vi "Weather Parse Test.vi"() -> ()   [LabVIEW 2020, in "CDM-Config.lvlib"] (continued)
        \"properties\": {\n                \"@id\": \"https://api.weather.gov/alerts/urn:oid:2.49.0.1.840.0.3fac73b358a1e250101ceb2ba749b5bee3a29f80.005.1\",\n                \"@type\": \"wx:Alert\",\n                \"id\": \"urn:oid:2.49.0.1.840.0.3fac73b358a1e250101ceb2ba749b5bee3a29f80.005.1\",\n                \"areaDesc\": \"Cape Cleare to Gore Point out to 15 NM\",\n                \"geocode\": {\n                    \"SAME\": [\n                        \"058715\"\n                    ],\n                    \"UGC\": [\n                        \"PKZ715\"\n                    ]\n                },\n                \"affectedZones\": [\n                    \"https://api.weather.gov/zones/forecast/PKZ715\"\n                ],\n                \"references\": [],\n                \"sent\": \"2025-12-03T04:02:00-09:00\",\n                \"effective\": \"2025-12-03T04:02:00-09:00\",\n                \"onset\": \"2025-12-03T04:00:00-09:00\",\n                \"expires\": \"2025-12-03T16:30:00-09:00\",\n                \"ends\": \"2025-12-04T05:00:00-09:00\",\n                \"status\": \"Actual\",\n                \"messageType\": \"Alert\",\n                \"category\": \"Met\",\n                \"severity\": \"Minor\",\n                \"certainty\": \"Likely\",\n                \"urgency\": \"Expected\",\n                \"event\": \"Small Craft Advisory\",\n                \"sender\": \"w-nws.webmaster@noaa.gov\",\n                \"senderName\": \"NWS Anchorage AK\",\n                \"headline\": \"Small Craft Advisory issued December 3 at 4:02AM AKST until December 4 at 5:00AM AKST by NWS Anchorage AK\",\n                \"description\": \"Coastal Waters Forecast for the Northern Gulf of Alaska Coast\\nup to 100 nm out including Kodiak Island and Cook Inlet.\\n\\nWind forecasts reflect the predominant speed and direction\\nexpected. Sea forecasts represent an average of the highest\\none-third of the combined wind wave and swell height.\\n\\n.TODAY...Variable wind 10 kt. Seas 8 ft. Rain.\\n.TONIGHT...Variable wind 10 kt. Seas 8 ft.\\n.THU...Variable wind 10 kt. Seas 7 ft.\\n.THU NIGHT...Variable wind 10 kt. Seas 6 ft.\\n.FRI...N wind 20 kt. Seas 5 ft.\\n.SAT THROUGH SUN...NE wind 25 kt. Seas 9 ft.\",\n                \"instruction\": null,\n                \"response\": \"Avoid\",\n                \"parameters\": {\n                    \"AWIPSidentifier\": [\n                        \"CWFAER\"\n                    ],\n                    \"WMOidentifier\": [\n                        \"FZAK51 PAFC 031302\"\n                    ],\n                    \"NWSheadline\": [\n                        \"SMALL CRAFT ADVISORY THROUGH TONIGHT\"\n                    ],\n                    \"BLOCKCHANNEL\": [\n                        \"EAS\",\n                        \"NWEM\",\n                        \"CMAS\"\n                    ],\n                    \"VTEC\": [\n                        \"/O.NEW.PAFC.SC.Y.9733.251203T1300Z-251204T1400Z/\"\n                    ],\n                    \"eventEndingTime\": [\n                        \"2025-12-04T05:00:00-09:00\"\n                    ]\n                },\n                \"scope\": \"Public\",\n                \"code\": \"IPAWSv1.0\",\n                \"language\": \"en-US\",\n                \"web\": \"http://www.weather.gov\",\n                \"eventCode\": {\n                    \"SAME\": [\n                        \"NWS\"\n                    ],\n                    \"NationalWeatherService\": [\n                        \"SCY\"\n                    ]\n                }\n            }\n        },\n        {\n            \"id\": \"https://api.weather.gov/alerts/urn:oid:2.49.0.1.840.0.3fac73b358a1e250101ceb2ba749b5bee3a29f80.004.1\",\n            \"type\": \"Feature\",\n            \"geometry\": null,\n            \"properties\": {\n                \"@id\": \"https://api.weather.gov/alerts/urn:oid:2.49.0.1.840.0.3fac73b358a1e250101ceb2ba749b5bee3a29f80.004.1\",\n                \"@type\": \"wx:Alert\",\n                \"id\": \"urn:oid:2.49.0.1.840.0.3fac73b358a1e250101ceb2ba749b5bee3a29f80.004.1\",\n                \"areaDesc\": \"Cape Suckling to Cape Cleare from 15 to 75 NM\",\n                \"geocode\": {\n                    \"SAME\": [\n                        \"058712\"\n                    ],\n                    \"UGC\": [\n                        \"PKZ712\"\n                    ]\n                },\n                \"affectedZones\": [\n                    \"https://api.weather.gov/zones/forecast/PKZ712\"\n                ],\n                \"references\": [],\n                \"sent\": \"2025-12-03T04:02:00-09:00\",\n                \"effective\": \"2025-12-03T04:02:00-09:00\",\n                \"onset\": \"2025-12-03T04:00:00-09:00\",\n                \"expires\": \"2025-12-03T16:30:00-09:00\",\n                \"ends\": \"2025-12-04T17:00:00-09:00\",\n                \"status\": \"Actual\",\n                \"messageType\": \"Alert\",\n                \"category\": \"Met\",\n                \"severity\": \"Minor\",\n                \"certainty\": \"Likely\",\n                \"urgency\": \"Expected\",\n                \"event\": \"Small Craft Advisory\",\n                \"sender\": \"w-nws.webmaster@noaa.gov\",\n                \"senderName\": \"NWS Anchorage AK\",\n                \"headline\": \"Small Craft Advisory issued December 3 at 4:02AM AKST until December 4 at 5:00PM AKST by NWS Anchorage AK\",\n                \"description\": \"Coastal Waters Forecast for the Northern Gulf of Alaska Coast\\nup to 100 nm out including Kodiak Island and Cook Inlet.\\n\\nWind forecasts reflect the predominant speed and direction\\nexpected. Sea forecasts represent an average of the highest\\none-third of the combined wind wave and swell height.\\n\\n.TODAY...S wind 15 kt. Seas 11 ft.\\n.TONIGHT...SW wind 15 kt. Seas 10 ft.\\n.THU...SW wind 15 kt. Seas 9 ft.\\n.THU NIGHT...Variable wind 10 kt. Seas 8 ft.\\n.FRI...N wind 15 kt. Seas 7 ft.\\n.SAT...SE wind 25 kt. Seas 9 ft.\\n.SUN...E wind 25 kt. Seas 13 ft.\",\n                \"instruction\": null,\n                \"response\": \"Avoid\",\n                \"parameters\": {\n                    \"AWIPSidentifier\": [\n                        \"CWFAER\"\n                    ],\n                    \"WMOidentifier\": [\n                        \"FZAK51 PAFC 031302\"\n                    ],\n                    \"NWSheadline\": [\n                        \"SMALL CRAFT ADVISORY THROUGH THURSDAY\"\n                    ],\n                    \"BLOCKCHANNEL\": [\n                        \"EAS\",\n                        \"NWEM\",\n                        \"CMAS\"\n                    ],\n                    \"VTEC\": [\n                        \"/O.NEW.PAFC.SC.Y.9732.251203T1300Z-251205T0200Z/\"\n                    ],\n                    \"eventEndingTime\": [\n                        \"2025-12-04T17:00:00-09:00\"\n                    ]\n                },\n                \"scope\": \"Public\",\n                \"code\": \"IPAWSv1.0\",\n                \"language\": \"en-US\",\n                \"web\": \"http://www.weather.gov\",\n                \"eventCode\": {\n                    \"SAME\": [\n                        \"NWS\"\n                    ],\n                    \"NationalWeatherService\": [\n                        \"SCY\"\n                    ]\n                }\n            }\n        },\n        {\n            \"id\": \"https://api.weather.gov/alerts/urn:oid:2.49.0.1.840.0.3fac73b358a1e250101ceb2ba749b5bee3a29f80.017.1\",\n            \"type\": \"Feature\",\n            \"geometry\": null,\n            \"properties\": {\n                \"@id\": \"https://api.weather.gov/alerts/urn:oid:2.49.0.1.840.0.3fac73b358a1e250101ceb2ba749b5bee3a29f80.017.1\",\n                \"@type\": \"wx:Alert\",\n                \"id\": \"urn:oid:2.49.0.1.840.0.3fac73b358a1e250101ceb2ba749b5bee3a29f80.017.1\",\n                \"areaDesc\": \"Gore Point to Marmot Island from 15 to 80 NM\",\n                \"geocode\": {\n                    \"SAME\": [\n                        \"058733\"\n                    ],\n                    \"UGC\": [\n                        \"PKZ733\"\n                    ]\n                },\n                \"affectedZones\": [\n                    \"https://api.weather.gov/zones/forecast/PKZ733\"\n                ],\n                \"references\": [],\n                \"sent\": \"2025-12-03T04:02:00-09:00\",\n                \"effective\": \"2025-12-03T04:02:00-09:00\",\n                \"onset\": \"2025-12-03T04:00:00-09:00\",\n                \"expires\": \"2025-12-03T16:30:00-09:00\",\n                \"ends\": \"2025-12-04T17:00:00-09:00\",\n                \"status\": \"Actual\",\n                \"messageType\": \"Alert\",\n                \"category\": \"Met\",\n                \"severity\": \"Minor\",\n                \"certainty\": \"Likely\",\n                \"urgency\": \"Expected\",\n                \"event\": \"Small Craft Advisory\",\n                \"sender\": \"w-nws.webmaster@noaa.gov\",\n                \"senderName\": \"NWS Anchorage AK\",\n                \"headline\": \"Small Craft Advisory issued December 3 at 4:02AM AKST until December 4 at 5:00PM AKST by NWS Anchorage AK\",\n                \"description\": \"Coastal Waters Forecast for the Northern Gulf of Alaska Coast\\nup to 100 nm out including Kodiak Island and Cook Inlet.\\n\\nWind forecasts reflect the predominant speed and direction\\nexpected. Sea forecasts represent an average of the highest\\none-third of the combined wind wave and swell height.\\n\\n.TODAY...SW wind 20 kt. Seas 11 ft.\\n.TONIGHT...SW wind 15 kt. Seas 10 ft.\\n.THU...S wind 15 kt. Seas 8 ft.\\n.THU NIGHT...Variable wind 10 kt. Seas 7 ft.\\n.FRI...N wind 25 kt. Seas 7 ft.\\n.SAT...N wind 25 kt. Seas 11 ft.\\n.SUN...NE wind 25 kt. Seas 16 ft.\",\n                \"instruction\": null,\n                \"response\": \"Avoid\",\n                \"parameters\": {\n                    \"AWIPSidentifier\": [\n                        \"CWFAER\"\n                    ],\n                    \"WMOidentifier\": [\n                        \"FZAK51 PAFC 031302\"\n                    ],\n                    \"NWSheadline\": [\n                        \"SMALL CRAFT ADVISORY THROUGH THURSDAY\"\n                    ],\n                    \"BLOCKCHANNEL\": [\n                        \"EAS\",\n                        \"NWEM\",\n                        \"CMAS\"\n                    ],\n                    \"VTEC\": [\n                        \"/O.NEW.PAFC.SC.Y.9735.251203T1300Z-251205T0200Z/\"\n                    ],\n                    \"eventEndingTime\": [\n                        \"2025-12-04T17:00:00-09:00\"\n                    ]\n                },\n                \"scope\": \"Public\",\n                \"code\": \"IPAWSv1.0\",\n                \"language\": \"en-US\",\n                \"web\": \"http://www.weather.gov\",\n                \"eventCode\": {\n                    \"SAME\": [\n                        \"NWS\"\n                    ],\n                    \"NationalWeatherService\": [\n                        \"SCY\"\n                    ]\n                }\n            }\n        },\n        {\n            \"id\": \"https://api.weather.gov/alerts/urn:oid:2.49.0.1.840.0.3fac73b358a1e250101ceb2ba749b5bee3a29f80.006.1\",\n            \"type\": \"Feature\",\n            \"geometry\": null,\n            \"properties\": {\n                \"@id\": \"https://api.weather.gov/alerts/urn:oid:2.49.0.1.840.0.3fac73b358a1e250101ceb2ba749b5bee3a29f80.006.1\",\n                \"@type\": \"wx:Alert\",\n                \"id\": \"urn:oid:2.49.0.1.840.0.3fac73b358a1e250101ceb2ba749b5bee3a29f80.006.1\",\n                \"areaDesc\": \"Cape Cleare to Gore Point from 15 to 75 NM\",\n                \"geocode\": {\n                    \"SAME\": [\n                        \"058716\"\n                    ],\n                    \"UGC\": [\n                        \"PKZ716\"\n                    ]\n                },\n                \"affectedZones\": [\n                    \"https://api.weather.gov/zones/forecast/PKZ716\"\n                ],\n                \"references\": [],\n                \"sent\": \"2025-12-03T04:02:00-09:00\",\n                \"effective\": \"2025-12-03T04:02:00-09:00\",\n                \"onset\": \"2025-12-03T04:00:00-09:00\",\n                \"expires\": \"2025-12-03T16:30:00-09:00\",\n                \"ends\": \"2025-12-04T17:00:00-09:00\",\n                \"status\": \"Actual\",\n                \"messageType\": \"Alert\",\n                \"category\": \"Met\",\n                \"severity\": \"Minor\",\n                \"certainty\": \"Likely\",\n                \"urgency\": \"Expected\",\n                \"event\": \"Small Craft Advisory\",\n                \"sender\": \"w-nws.webmaster@noaa.gov\",\n                \"senderName\": \"NWS Anchorage AK\",\n                \"headline\": \"Small Craft Advisory issued December 3 at 4:02AM AKST until December 4 at 5:00PM AKST by NWS Anchorage AK\",\n                \"description\": \"Coastal Waters Forecast for the Northern Gulf of Alaska Coast\\nup to 100 nm out including Kodiak Island and Cook Inlet.\\n\\nWind forecasts reflect the predominant speed and direction\\nexpected. Sea forecasts represent an average of the highest\\none-third of the combined wind wave and swell height.\\n\\n.TODAY...SW wind 15 kt. Seas 10 ft.\\n.TONIGHT...SW wind 15 kt. Seas 10 ft.\\n.THU...SW wind 15 kt. Seas 8 ft.\\n.THU NIGHT...Variable wind 10 kt. Seas 7 ft.\\n.FRI...N wind 15 kt. Seas 7 ft.\\n.SAT...NE wind 25 kt. Seas 11 ft.\\n.SUN...NE wind 25 kt. Seas 15 ft.\",\n                \"instruction\": null,\n                \"response\": \"Avoid\",\n                \"parameters\": {\n                    \"AWIPSidentifier\": [\n                        \"CWFAER\"\n                    ],\n                    \"WMOidentifier\": [\n                        \"FZAK51 PAFC 031302\"\n                    ],\n                    \"NWSheadline\": [\n                        \"SMALL CRAFT ADVISORY THROUGH THURSDAY\"\n                    ],\n                    \"BLOCKCHANNEL\": [\n                        \"EAS\",\n                        \"NWEM\",\n                        \"CMAS\"\n                    ],\n                    \"VTEC\": [\n                        \"/O.NEW.PAFC.SC.Y.9734.251203T1300Z-251205T0200Z/\"\n                    ],\n                    \"eventEndingTime\": [\n                        \"2025-12-04T17:00:00-09:00\"\n                    ]\n                },\n                \"scope\": \"Public\",\n                \"code\": \"IPAWSv1.0\",\n                \"language\": \"en-US\",\n                \"web\": \"http://www.weather.gov\",\n                \"eventCode\": {\n                    \"SAME\": [\n                        \"NWS\"\n                    ],\n                    \"NationalWeatherService\": [\n                        \"SCY\"\n                    ]\n                }\n            }\n        },\n        {\n            \"id\": \"https://api.weather.gov/alerts/urn:oid:2.49.0.1.840.0.3fac73b358a1e250101ceb2ba749b5bee3a29f80.002.1\",\n            \"type\": \"Feature\",\n            \"geometry\": null,\n            \"properties\": {\n                \"@id\": \"https://api.weather.gov/alerts/urn:oid:2.49.0.1.840.0.3fac73b358a1e250101ceb2ba749b5bee3a29f80.002.1\",\n                \"@type\": \"wx:Alert\",\n                \"id\": \"urn:oid:2.49.0.1.840.0.3fac73b358a1e250101ceb2ba749b5bee3a29f80.002.1\",\n                \"areaDesc\": \"Cape Suckling to Gravel Point out to 15 NM\",\n                \"geocode\": {\n                    \"SAME\": [\n                        \"058710\"\n                    ],\n                    \"UGC\": [\n                        \"PKZ710\"\n                    ]\n                },\n                \"affectedZones\": [\n                    \"https://api.weather.gov/zones/forecast/PKZ710\"\n                ],\n                \"references\": [],\n                \"sent\": \"2025-12-03T04:02:00-09:00\",\n                \"effective\": \"2025-12-03T04:02:00-09:00\",\n                \"onset\": \"2025-12-03T04:00:00-09:00\",\n                \"expires\": \"2025-12-03T16:30:00-09:00\",\n                \"ends\": \"2025-12-04T17:00:00-09:00\",\n                \"status\": \"Actual\",\n                \"messageType\": \"Alert\",\n                \"category\": \"Met\",\n                \"severity\": \"Minor\",\n                \"certainty\": \"Likely\",\n                \"urgency\": \"Expected\",\n                \"event\": \"Small Craft Advisory\",\n                \"sender\": \"w-nws.webmaster@noaa.gov\",\n                \"senderName\": \"NWS Anchorage AK\",\n                \"headline\": \"Small Craft Advisory issued December 3 at 4:02AM AKST until December 4 at 5:00PM AKST by NWS Anchorage AK\",\n                \"description\": \"Coastal Waters Forecast for the Northern Gulf of Alaska Coast\\nup to 100 nm out including Kodiak Island and Cook Inlet.\\n\\nWind forecasts reflect the predominant speed and direction\\nexpected. Sea forecasts represent an average of the highest\\none-third of the combined wind wave and swell height.\\n\\n.TODAY...SE wind 25 kt becoming S 15 kt in the afternoon.\\nSeas 10 ft. Rain.\\n.TONIGHT...SW wind 15 kt. Seas 9 ft.\\n.THU...Variable wind 10 kt. Seas 8 ft.\\n.THU NIGHT...Variable wind 10 kt. Seas 7 ft.\\n.FRI...NE wind 25 kt. Seas 6 ft.\\n.SAT THROUGH SUN...NE wind 30 kt. Seas 9 ft.\",\n                \"instruction\": null,\n                \"response\": \"Avoid\",\n                \"parameters\": {\n                    \"AWIPSidentifier\": [\n                        \"CWFAER\"\n                    ],\n                    \"WMOidentifier\": [\n                        \"FZAK51 PAFC 031302\"\n                    ],\n                    \"NWSheadline\": [\n                        \"SMALL CRAFT ADVISORY THROUGH THURSDAY\"\n                    ],\n                    \"BLOCKCHANNEL\": [\n                        \"EAS\",\n                        \"NWEM\",\n                        \"CMAS\"\n                    ],\n                    \"VTEC\": [\n                        \"/O.NEW.PAFC.SC.Y.9730.251203T1300Z-251205T0200Z/\"\n                    ],\n                    \"eventEndingTime\": [\n                        \"2025-12-04T17:00:00-09:00\"\n                    ]\n                },\n                \"scope\": \"Public\",\n                \"code\": \"IPAWSv1.0\",\n                \"language\": \"en-US\",\n                \"web\": \"http://www.weather.gov\",\n                \"eventCode\": {\n                    \"SAME\": [\n                        \"NWS\"\n                    ],\n                    \"NationalWeatherService\": [\n                        \"SCY\"\n                    ]\n                }\n            }\n        },\n        {\n            \"id\": \"https://api.weather.gov/alerts/urn:oid:2.49.0.1.840.0.16ee1729296b80b5948b72c512c8722f6075ae6c.004.1\",\n            \"type\": \"Feature\",\n            \"geometry\": null,\n            \"properties\": {\n                \"@id\": \"https://api.weather.gov/alerts/urn:oid:2.49.0.1.840.0.16ee1729296b80b5948b72c512c8722f6075ae6c.004.1\",\n                \"@type\": \"wx:Alert\",\n                \"id\": \"urn:oid:2.49.0.1.840.0.16ee1729296b80b5948b72c512c8722f6075ae6c.004.1\",\n                \"areaDesc\": \"Castle Cape to Cape Tolstoi out to 15 NM\",\n                \"geocode\": {\n                    \"SAME\": [\n                        \"058752\"\n                    ],\n                    \"UGC\": [\n                        \"PKZ752\"\n                    ]\n                },\n                \"affectedZones\": [\n                    \"https://api.weather.gov/zones/forecast/PKZ752\"\n                ],\n                \"references\": [],\n                \"sent\": \"2025-12-03T04:00:00-09:00\",\n                \"effective\": \"2025-12-03T04:00:00-09:00\",\n                \"onset\": \"2025-12-03T04:00:00-09:00\",\n                \"expires\": \"2025-12-03T17:00:00-09:00\",\n                \"ends\": \"2025-12-04T17:00:00-09:00\",\n                \"status\": \"Actual\",\n                \"messageType\": \"Alert\",\n                \"category\": \"Met\",\n                \"severity\": \"Minor\",\n                \"certainty\": \"Likely\",\n                \"urgency\": \"Expected\",\n                \"event\": \"Small Craft Advisory\",\n                \"sender\": \"w-nws.webmaster@noaa.gov\",\n                \"senderName\": \"NWS Anchorage AK\",\n                \"headline\": \"Small Craft Advisory issued December 3 at 4:00AM AKST until December 4 at 5:00PM AKST by NWS Anchorage AK\",\n                \"description\": \"Coastal Waters Forecast for Southwest Alaska+Bristol Bay+The\\nAlaska Peninsula Waters and the Aleutian Islands up to 100 nm out.\\n\\nWind forecasts reflect the predominant speed and direction\\nexpected. Sea forecasts represent an average of the highest\\none-third of the combined wind wave and swell height.\\n\\n.TODAY...SE wind 20 kt. Seas 9 ft. Rain showers.\\n.TONIGHT...SE wind 20 kt. Seas 9 ft. Rain showers.\\n.THU...SE wind 15 kt. Seas 8 ft. Rain showers.\\n.THU NIGHT...NE wind 20 kt. Seas 6 ft.\\n.FRI...N wind 20 kt. Seas 5 ft.\\n.SAT...NW wind 35 kt. Seas 5 ft.\\n.SUN...N wind 20 kt. Seas 2 ft.\",\n                \"instruction\": null,\n                \"response\": \"Avoid\",\n                \"parameters\": {\n                    \"AWIPSidentifier\": [\n                        \"CWFALU\"\n                    ],\n                    \"WMOidentifier\": [\n                        \"FZAK52 PAFC 031300\"\n                    ],\n                    \"NWSheadline\": [\n                        \"SMALL CRAFT ADVISORY THROUGH THURSDAY\"\n                    ],\n                    \"BLOCKCHANNEL\": [\n                        \"EAS\",\n                        \"NWEM\",\n                        \"CMAS\"\n                    ],\n                    \"VTEC\": [\n                        \"/O.NEW.PAFC.SC.Y.5640.251203T1300Z-251205T0200Z/\"\n                    ],\n                    \"eventEndingTime\": [\n                        \"2025-12-04T17:00:00-09:00\"\n                    ]\n                },\n                \"scope\": \"Public\",\n                \"code\": \"IPAWSv1.0\",\n                \"language\": \"en-US\",\n                \"web\": \"http://www.weather.gov\",\n                \"eventCode\": {\n                    \"SAME\": [\n                        \"NWS\"\n                    ],\n                    \"NationalWeatherService\": [\n                        \"SCY\"\n                    ]\n                }\n            }\n        },\n        {\n            \"id\": \"https://api.weather.gov/alerts/urn:oid:2.49.0.1.840.0.16ee1729296b80b5948b72c512c8722f6075ae6c.003.1\",\n            \"type\": \"Feature\",\n            \"geometry\": null,\n            \"properties\": {\n                \"@id\": \"https://api.weather.gov/alerts/urn:oid:2.49.0.1.840.0.16ee1729296b80b5948b72c512c8722f6075ae6c.003.1\",\n                \"@type\": \"wx:Alert\",\n                \"id\": \"urn:oid:2.49.0.1.840.0.16ee1729296b80b5948b72c512c8722f6075ae6c.003.1\",\n                \"areaDesc\": \"Sitkinak to Castle Cape from 15 to 100 NM\",\n                \"geocode\": {\n                    \"SAME\": [\n                        \"058751\"\n                    ],\n                    \"UGC\": [\n                        \"PKZ751\"\n                    ]\n                },\n                \"affectedZones\": [\n                    \"https://api.weather.gov/zones/forecast/PKZ751\"\n                ],\n                \"references\": [],\n                \"sent\": \"2025-12-03T04:00:00-09:00\",\n                \"effective\": \"2025-12-03T04:00:00-09:00\",\n                \"onset\": \"2025-12-03T04:00:00-09:00\",\n                \"expires\": \"2025-12-03T17:00:00-09:00\",\n                \"ends\": \"2025-12-04T17:00:00-09:00\",\n                \"status\": \"Actual\",\n                \"messageType\": \"Alert\",\n                \"category\": \"Met\",\n                \"severity\": \"Minor\",\n                \"certainty\": \"Likely\",\n                \"urgency\": \"Expected\",\n                \"event\": \"Small Craft Advisory\",\n                \"sender\": \"w-nws.webmaster@noaa.gov\",\n                \"senderName\": \"NWS Anchorage AK\",\n                \"headline\": \"Small Craft Advisory issued December 3 at 4:00AM AKST until December 4 at 5:00PM AKST by NWS Anchorage AK\",\n                \"description\": \"Coastal Waters Forecast for Southwest Alaska+Bristol Bay+The\\nAlaska Peninsula Waters and the Aleutian Islands up to 100 nm out.\\n\\nWind forecasts reflect the predominant speed and direction\\nexpected. Sea forecasts represent an average of the highest\\none-third of the combined wind wave and swell height.\\n\\n.TODAY...S wind 25 kt. Seas 14 ft.\\n.TONIGHT...S wind 25 kt. Seas 14 ft.\\n.THU...SE wind 20 kt. Seas 12 ft.\\n.THU NIGHT...NE wind 20 kt. Seas 8 ft.\\n.FRI THROUGH SAT...NW wind 35 kt. Seas 10 ft.\\n.SUN...NW wind 25 kt. Seas 9 ft.\",\n                \"instruction\": null,\n                \"response\": \"Avoid\",\n                \"parameters\": {\n                    \"AWIPSidentifier\": [\n                        \"CWFALU\"\n                    ],\n                    \"WMOidentifier\": [\n                        \"FZAK52 PAFC 031300\"\n                    ],\n                    \"NWSheadline\": [\n                        \"SMALL CRAFT ADVISORY THROUGH THURSDAY\"\n                    ],\n                    \"BLOCKCHANNEL\": [\n                        \"EAS\",\n                        \"NWEM\",\n                        \"CMAS\"\n                    ],\n                    \"VTEC\": [\n                        \"/O.NEW.PAFC.SC.Y.5639.251203T1300Z-251205T0200Z/\"\n                    ],\n                    \"eventEndingTime\": [\n                        \"2025-12-04T17:00:00-09:00\"\n                    ]\n                },\n                \"scope\": \"Public\",\n                \"code\": \"IPAWSv1.0\",\n                \"language\": \"en-US\",\n                \"web\": \"http://www.weather.gov\",\n                \"eventCode\": {\n                    \"SAME\": [\n                        \"NWS\"\n                    ],\n                    \"NationalWeatherService\": [\n                        \"SCY\"\n                    ]\n                }\n            }\n        },\n        {\n            \"id\": \"https://api.weather.gov/alerts/urn:oid:2.49.0.1.840.0.16ee1729296b80b5948b72c512c8722f6075ae6c.007.1\",\n            \"type\": \"Feature\",\n            \"geometry\": null,\n            \"properties\": {\n                \"@id\": \"https://api.weather.gov/alerts/urn:oid:2.49.0.1.840.0.16ee1729296b80b5948b72c512c8722f6075ae6c.007.1\",\n                \"@type\": \"wx:Alert\",\n                \"id\": \"urn:oid:2.49.0.1.840.0.16ee1729296b80b5948b72c512c8722f6075ae6c.007.1\",\n                \"areaDesc\": \"Cape Tolstoi to Cape Sarichef from 15 to 100 NM\",\n                \"geocode\": {\n                    \"SAME\": [\n                        \"058755\"\n                    ],\n                    \"UGC\": [\n                        \"PKZ755\"\n                    ]\n                },\n                \"affectedZones\": [\n                    \"https://api.weather.gov/zones/forecast/PKZ755\"\n                ],\n                \"references\": [],\n                \"sent\": \"2025-12-03T04:00:00-09:00\",\n                \"effective\": \"2025-12-03T04:00:00-09:00\",\n                \"onset\": \"2025-12-03T04:00:00-09:00\",\n                \"expires\": \"2025-12-03T17:00:00-09:00\",\n                \"ends\": \"2025-12-04T17:00:00-09:00\",\n                \"status\": \"Actual\",\n                \"messageType\": \"Alert\",\n                \"category\": \"Met\",\n                \"severity\": \"Minor\",\n                \"certainty\": \"Likely\",\n                \"urgency\": \"Expected\",\n                \"event\": \"Small Craft Advisory\",\n                \"sender\": \"w-nws.webmaster@noaa.gov\",\n                \"senderName\": \"NWS Anchorage AK\",\n                \"headline\": \"Small Craft Advisory issued December 3 at 4:00AM AKST until December 4 at 5:00PM AKST by NWS Anchorage AK\",\n                \"description\": \"Coastal Waters Forecast for Southwest Alaska+Bristol Bay+The\\nAlaska Peninsula Waters and the Aleutian Islands up to 100 nm out.\\n\\nWind forecasts reflect the predominant speed and direction\\nexpected. Sea forecasts represent an average of the highest\\none-third of the combined wind wave and swell height.\\n\\n.TODAY...SE wind 30 kt. Seas 17 ft. Rain showers.\\n.TONIGHT...SE wind 20 kt. Seas 14 ft.\\n.THU...SE wind 15 kt. Seas 11 ft.\\n.THU NIGHT...E wind 15 kt. Seas 7 ft.\\n.FRI...NW wind 25 kt. Seas 5 ft.\\n.SAT...NW wind 35 kt. Seas 13 ft.\\n.SUN...N wind 25 kt. Seas 10 ft.\",\n                \"instruction\": null,\n                \"response\": \"Avoid\",\n                \"parameters\": {\n                    \"AWIPSidentifier\": [\n                        \"CWFALU\"\n                    ],\n                    \"WMOidentifier\": [\n                        \"FZAK52 PAFC 031300\"\n                    ],\n                    \"NWSheadline\": [\n                        \"SMALL CRAFT ADVISORY THROUGH THURSDAY\"\n                    ],\n                    \"BLOCKCHANNEL\": [\n                        \"EAS\",\n                        \"NWEM\",\n                        \"CMAS\"\n                    ],\n                    \"VTEC\": [\n                        \"/O.NEW.PAFC.SC.Y.5643.251203T1300Z-251205T0200Z/\"\n                    ],\n                    \"eventEndingTime\": [\n                        \"2025-12-04T17:00:00-09:00\"\n                    ]\n                },\n                \"scope\": \"Public\",\n                \"code\": \"IPAWSv1.0\",\n                \"language\": \"en-US\",\n                \"web\": \"http://www.weather.gov\",\n                \"eventCode\": {\n                    \"SAME\": [\n                        \"NWS\"\n                    ],\n                    \"NationalWeatherService\": [\n                        \"SCY\"\n                    ]\n                }\n            }\n        },\n        {\n            \"id\": \"https://api.weather.gov/alerts/urn:oid:2.49.0.1.840.0.16ee1729296b80b5948b72c512c8722f6075ae6c.006.1\",\n            \"type\": \"Feature\",\n            \"geometry\": null,\n            \"properties\": {\n                \"@id\": \"https://api.weather.gov/alerts/urn:oid:2.49.0.1.840.0.16ee1729296b80b5948b72c512c8722f6075ae6c.006.1\",\n                \"@type\": \"wx:Alert\",\n                \"id\": \"urn:oid:2.49.0.1.840.0.16ee1729296b80b5948b72c512c8722f6075ae6c.006.1\",\n                \"areaDesc\": \"Cape Tolstoi to Cape Sarichef out to 15 NM\",\n                \"geocode\": {\n                    \"SAME\": [\n                        \"058754\"\n                    ],\n                    \"UGC\": [\n                        \"PKZ754\"\n                    ]\n                },\n                \"affectedZones\": [\n                    \"https://api.weather.gov/zones/forecast/PKZ754\"\n                ],\n                \"references\": [],\n                \"sent\": \"2025-12-03T04:00:00-09:00\",\n                \"effective\": \"2025-12-03T04:00:00-09:00\",\n                \"onset\": \"2025-12-03T04:00:00-09:00\",\n                \"expires\": \"2025-12-03T17:00:00-09:00\",\n                \"ends\": \"2025-12-04T17:00:00-09:00\",\n                \"status\": \"Actual\",\n                \"messageType\": \"Alert\",\n                \"category\": \"Met\",\n                \"severity\": \"Minor\",\n                \"certainty\": \"Likely\",\n                \"urgency\": \"Expected\",\n                \"event\": \"Small Craft Advisory\",\n                \"sender\": \"w-nws.webmaster@noaa.gov\",\n                \"senderName\": \"NWS Anchorage AK\",\n                \"headline\": \"Small Craft Advisory issued December 3 at 4:00AM AKST until December 4 at 5:00PM AKST by NWS Anchorage AK\",\n                \"description\": \"Coastal Waters Forecast for Southwest Alaska+Bristol Bay+The\\nAlaska Peninsula Waters and the Aleutian Islands up to 100 nm out.\\n\\nWind forecasts reflect the predominant speed and direction\\nexpected. Sea forecasts represent an average of the highest\\none-third of the combined wind wave and swell height.\\n\\n.TODAY...E wind 25 kt. Seas 13 ft. Rain showers.\\n.TONIGHT...Variable wind 10 kt. Seas 10 ft.\\n.THU...NE wind 15 kt. Seas 8 ft.\\n.THU NIGHT...NE wind 15 kt. Seas 6 ft.\\n.FRI...N wind 30 kt. Seas 5 ft.\\n.SAT...NW wind 35 kt. Seas 6 ft.\\n.SUN...N wind 25 kt. Seas 5 ft.\",\n                \"instruction\": null,\n                \"response\": \"Avoid\",\n                \"parameters\": {\n                    \"AWIPSidentifier\": [\n                        \"CWFALU\"\n                    ],\n                    \"WMOidentifier\": [\n                        \"FZAK52 PAFC 031300\"\n                    ],\n                    \"NWSheadline\": [\n                        \"SMALL CRAFT ADVISORY THROUGH THURSDAY\"\n                    ],\n                    \"BLOCKCHANNEL\": [\n                        \"EAS\",\n                        \"NWEM\",\n                        \"CMAS\"\n                    ],\n                    \"VTEC\": [\n                        \"/O.NEW.PAFC.SC.Y.5642.251203T1300Z-251205T0200Z/\"\n                    ],\n                    \"eventEndingTime\": [\n                        \"2025-12-04T17:00:00-09:00\"\n                    ]\n                },\n                \"scope\": \"Public\",\n                \"code\": \"IPAWSv1.0\",\n                \"language\": \"en-US\",\n                \"web\": \"http://www.weather.gov\",\n                \"eventCode\": {\n                    \"SAME\": [\n                        \"NWS\"\n                    ],\n                    \"NationalWeatherService\": [\n                        \"SCY\"\n                    ]\n                }\n            }\n        },\n        {\n            \"id\": \"https://api.weather.gov/alerts/urn:oid:2.49.0.1.840.0.16ee1729296b80b5948b72c512c8722f6075ae6c.005.1\",\n            \"type\": \"Feature\",\n            \"geometry\": null,\n            \"properties\": {\n                \"@id\": \"https://api.weather.gov/alerts/urn:oid:2.49.0.1.840.0.16ee1729296b80b5948b72c512c8722f6075ae6c.005.1\",\n                \"@type\": \"wx:Alert\",\n                \"id\": \"urn:oid:2.49.0.1.840.0.16ee1729296b80b5948b72c512c8722f6075ae6c.005.1\",\n                \"areaDesc\": \"Castle Cape to Cape Tolstoi from 15 to 100 NM\",\n                \"geocode\": {\n                    \"SAME\": [\n                        \"058753\"\n                    ],\n                    \"UGC\": [\n                        \"PKZ753\"\n                    ]\n                },\n                \"affectedZones\": [\n                    \"https://api.weather.gov/zones/forecast/PKZ753\"\n                ],\n                \"references\": [],\n                \"sent\": \"2025-12-03T04:00:00-09:00\",\n                \"effective\": \"2025-12-03T04:00:00-09:00\",\n                \"onset\": \"2025-12-03T04:00:00-09:00\",\n                \"expires\": \"2025-12-03T17:00:00-09:00\",\n                \"ends\": \"2025-12-04T17:00:00-09:00\",\n                \"status\": \"Actual\",\n                \"messageType\": \"Alert\",\n                \"category\": \"Met\",\n                \"severity\": \"Minor\",\n                \"certainty\": \"Likely\",\n                \"urgency\": \"Expected\",\n                \"event\": \"Small Craft Advisory\",\n                \"sender\": \"w-nws.webmaster@noaa.gov\",\n                \"senderName\": \"NWS Anchorage AK\",\n                \"headline\": \"Small Craft Advisory issued December 3 at 4:00AM AKST until December 4 at 5:00PM AKST by NWS Anchorage AK\",\n                \"description\": \"Coastal Waters Forecast for Southwest Alaska+Bristol Bay+The\\nAlaska Peninsula Waters and the Aleutian Islands up to 100 nm out.\\n\\nWind forecasts reflect the predominant speed and direction\\nexpected. Sea forecasts represent an average of the highest\\none-third of the combined wind wave and swell height.\\n\\n.TODAY...SE wind 30 kt. Seas 17 ft. Rain showers.\\n.TONIGHT...S wind 20 kt. Seas 15 ft. Rain showers.\\n.THU...SE wind 20 kt. Seas 12 ft.\\n.THU NIGHT...NE wind 20 kt. Seas 8 ft.\\n.FRI...NW wind 20 kt. Seas 6 ft.\\n.SAT...NW wind 35 kt. Seas 13 ft.\\n.SUN...N wind 25 kt. Seas 11 ft.\",\n                \"instruction\": null,\n                \"response\": \"Avoid\",\n                \"parameters\": {\n                    \"AWIPSidentifier\": [\n                        \"CWFALU\"\n                    ],\n                    \"WMOidentifier\": [\n                        \"FZAK52 PAFC 031300\"\n                    ],\n                    \"NWSheadline\": [\n                        \"SMALL CRAFT ADVISORY THROUGH THURSDAY\"\n                    ],\n                    \"BLOCKCHANNEL\": [\n                        \"EAS\",\n                        \"NWEM\",\n                        \"CMAS\"\n                    ],\n                    \"VTEC\": [\n                        \"/O.NEW.PAFC.SC.Y.5641.251203T1300Z-251205T0200Z/\"\n                    ],\n                    \"eventEndingTime\": [\n                        \"2025-12-04T17:00:00-09:00\"\n                    ]\n                },\n                \"scope\": \"Public\",\n                \"code\": \"IPAWSv1.0\",\n                \"language\": \"en-US\",\n                \"web\": \"http://www.weather.gov\",\n                \"eventCode\": {\n                    \"SAME\": [\n                        \"NWS\"\n                    ],\n                    \"NationalWeatherService\": [\n                        \"SCY\"\n                    ]\n                }\n            }\n        },\n        {\n            \"id\": \"https://api.weather.gov/alerts/urn:oid:2.49.0.1.840.0.16ee1729296b80b5948b72c512c8722f6075ae6c.023.1\",\n            \"type\": \"Feature\",\n            \"geometry\": null,\n            \"properties\": {\n                \"@id\": \"https://api.weather.gov/alerts/urn:oid:2.49.0.1.840.0.16ee1729296b80b5948b72c512c8722f6075ae6c.023.1\",\n                \"@type\": \"wx:Alert\",\n                \"id\": \"urn:oid:2.49.0.1.840.0.16ee1729296b80b5948b72c512c8722f6075ae6c.023.1\",\n                \"areaDesc\": \"Seguam to Adak Pacific Side out to 15 NM\",\n                \"geocode\": {\n                    \"SAME\": [\n                        \"058782\"\n                    ],\n                    \"UGC\": [\n                        \"PKZ782\"\n                    ]\n                },\n                \"affectedZones\": [\n                    \"https://api.weather.gov/zones/forecast/PKZ782\"\n                ],\n                \"references\": [],\n                \"sent\": \"2025-12-03T04:00:00-09:00\",\n                \"effective\": \"2025-12-03T04:00:00-09:00\",\n                \"onset\": \"2025-12-03T04:00:00-09:00\",\n                \"expires\": \"2025-12-03T17:00:00-09:00\",\n                \"ends\": \"2025-12-04T05:00:00-09:00\",\n                \"status\": \"Actual\",\n                \"messageType\": \"Alert\",\n                \"category\": \"Met\",\n                \"severity\": \"Moderate\",\n                \"certainty\": \"Likely\",\n                \"urgency\": \"Expected\",\n                \"event\": \"Gale Warning\",\n                \"sender\": \"w-nws.webmaster@noaa.gov\",\n                \"senderName\": \"NWS Anchorage AK\",\n                \"headline\": \"Gale Warning issued December 3 at 4:00AM AKST until December 4 at 5:00AM AKST by NWS Anchorage AK\",\n                \"description\": \"Coastal Waters Forecast for Southwest Alaska+Bristol Bay+The\\nAlaska Peninsula Waters and the Aleutian Islands up to 100 nm out.\\n\\nWind forecasts reflect the predominant speed and direction\\nexpected. Sea forecasts represent an average of the highest\\none-third of the combined wind wave and swell height.\\n\\n.TODAY...N wind 40 kt. Seas 14 ft. Rain.\\n.TONIGHT...N wind 35 kt. Seas 12 ft.\\n.THU...N wind 25 kt diminishing to 15 kt in the afternoon. Seas\\n8 ft.\\n.THU NIGHT...NE wind 15 kt. Seas 5 ft.\\n.FRI...E wind 15 kt. Seas 10 ft.\\n.SAT THROUGH SUN...N wind 25 kt. Seas 11 ft.\",\n                \"instruction\": null,\n                \"response\": \"Avoid\",\n                \"parameters\": {\n                    \"AWIPSidentifier\": [\n                        \"CWFALU\"\n                    ],\n                    \"WMOidentifier\": [\n                        \"FZAK52 PAFC 031300\"\n                    ],\n                    \"NWSheadline\": [\n                        \"GALE WARNING THROUGH TONIGHT\"\n                    ],\n                    \"BLOCKCHANNEL\": [\n                        \"EAS\",\n                        \"NWEM\",\n                        \"CMAS\"\n                    ],\n                    \"VTEC\": [\n                        \"/O.NEW.PAFC.GL.W.5658.251203T1300Z-251204T1400Z/\"\n                    ],\n                    \"eventEndingTime\": [\n                        \"2025-12-04T05:00:00-09:00\"\n                    ]\n                },\n                \"scope\": \"Public\",\n                \"code\": \"IPAWSv1.0\",\n                \"language\": \"en-US\",\n                \"web\": \"http://www.weather.gov\",\n                \"eventCode\": {\n                    \"SAME\": [\n                        \"NWS\"\n                    ],\n                    \"NationalWeatherService\": [\n                        \"GLW\"\n                    ]\n                }\n            }\n        },\n        {\n            \"id\": \"https://api.weather.gov/alerts/urn:oid:2.49.0.1.840.0.16ee1729296b80b5948b72c512c8722f6075ae6c.022.1\",\n            \"type\": \"Feature\",\n            \"geometry\": null,\n            \"properties\": {\n                \"@id\": \"https://api.weather.gov/alerts/urn:oid:2.49.0.1.840.0.16ee1729296b80b5948b72c512c8722f6075ae6c.022.1\",\n                \"@type\": \"wx:Alert\",\n                \"id\": \"urn:oid:2.49.0.1.840.0.16ee1729296b80b5948b72c512c8722f6075ae6c.022.1\",\n                \"areaDesc\": \"Seguam to Adak Bering Side from 15 to 85 NM\",\n                \"geocode\": {\n                    \"SAME\": [\n                        \"058781\"\n                    ],\n                    \"UGC\": [\n                        \"PKZ781\"\n                    ]\n                },\n                \"affectedZones\": [\n                    \"https://api.weather.gov/zones/forecast/PKZ781\"\n                ],\n                \"references\": [],\n                \"sent\": \"2025-12-03T04:00:00-09:00\",\n                \"effective\": \"2025-12-03T04:00:00-09:00\",\n                \"onset\": \"2025-12-03T04:00:00-09:00\",\n                \"expires\": \"2025-12-03T17:00:00-09:00\",\n                \"ends\": \"2025-12-04T05:00:00-09:00\",\n                \"status\": \"Actual\",\n                \"messageType\": \"Alert\",\n                \"category\": \"Met\",\n                \"severity\": \"Moderate\",\n                \"certainty\": \"Likely\",\n                \"urgency\": \"Expected\",\n                \"event\": \"Gale Warning\",\n                \"sender\": \"w-nws.webmaster@noaa.gov\",\n                \"senderName\": \"NWS Anchorage AK\",\n                \"headline\": \"Gale Warning issued December 3 at 4:00AM AKST until December 4 at 5:00AM AKST by NWS Anchorage AK\",\n                \"description\": \"Coastal Waters Forecast for Southwest Alaska+Bristol Bay+The\\nAlaska Peninsula Waters and the Aleutian Islands up to 100 nm out.\\n\\nWind forecasts reflect the predominant speed and direction\\nexpected. Sea forecasts represent an average of the highest\\none-third of the combined wind wave and swell height.\\n\\n.TODAY...N wind 40 kt. Seas 28 ft. Rain.\\n.TONIGHT...N wind 35 kt. Seas 23 ft.\\n.THU...NE wind 25 kt. Seas 16 ft.\\n.THU NIGHT...E wind 15 kt. Seas 10 ft.\\n.FRI...E wind 15 kt. Seas 7 ft.\\n.SAT...NE wind 25 kt. Seas 9 ft.\\n.SUN...N wind 30 kt. Seas 22 ft.\",\n                \"instruction\": null,\n                \"response\": \"Avoid\",\n                \"parameters\": {\n                    \"AWIPSidentifier\": [\n                        \"CWFALU\"\n                    ],\n                    \"WMOidentifier\": [\n                        \"FZAK52 PAFC 031300\"\n                    ],\n                    \"NWSheadline\": [\n                        \"GALE WARNING THROUGH TONIGHT\"\n                    ],\n                    \"BLOCKCHANNEL\": [\n                        \"EAS\",\n                        \"NWEM\",\n                        \"CMAS\"\n                    ],\n                    \"VTEC\": [\n                        \"/O.NEW.PAFC.GL.W.5657.251203T1300Z-251204T1400Z/\"\n                    ],\n                    \"eventEndingTime\": [\n                        \"2025-12-04T05:00:00-09:00\"\n                    ]\n                },\n                \"scope\": \"Public\",\n                \"code\": \"IPAWSv1.0\",\n                \"language\": \"en-US\",\n                \"web\": \"http://www.weather.gov\",\n                \"eventCode\": {\n                    \"SAME\": [\n                        \"NWS\"\n                    ],\n                    \"NationalWeatherService\": [\n                        \"GLW\"\n                    ]\n                }\n            }\n        },\n        {\n            \"id\": \"https://api.weather.gov/alerts/urn:oid:2.49.0.1.840.0.16ee1729296b80b5948b72c512c8722f6075ae6c.025.1\",\n            \"type\": \"Feature\",\n            \"geometry\": null,\n            \"properties\": {\n                \"@id\": \"https://api.weather.gov/alerts/urn:oid:2.49.0.1.840.0.16ee1729296b80b5948b72c512c8722f6075ae6c.025.1\",\n                \"@type\": \"wx:Alert\",\n                \"id\": \"urn:oid:2.49.0.1.840.0.16ee1729296b80b5948b72c512c8722f6075ae6c.025.1\",\n                \"areaDesc\": \"Adak to Kiska Bering Side\",\n                \"geocode\": {\n                    \"SAME\": [\n                        \"058784\"\n                    ],\n                    \"UGC\": [\n                        \"PKZ784\"\n                    ]\n                },\n                \"affectedZones\": [\n                    \"https://api.weather.gov/zones/forecast/PKZ784\"\n                ],\n                \"references\": [],\n                \"sent\": \"2025-12-03T04:00:00-09:00\",\n                \"effective\": \"2025-12-03T04:00:00-09:00\",\n                \"onset\": \"2025-12-03T05:00:00-09:00\",\n                \"expires\": \"2025-12-03T17:00:00-09:00\",\n                \"ends\": \"2025-12-03T17:00:00-09:00\",\n                \"status\": \"Actual\",\n                \"messageType\": \"Alert\",\n                \"category\": \"Met\",\n                \"severity\": \"Moderate\",\n                \"certainty\": \"Likely\",\n                \"urgency\": \"Expected\",\n                \"event\": \"Gale Warning\",\n                \"sender\": \"w-nws.webmaster@noaa.gov\",\n                \"senderName\": \"NWS Anchorage AK\",\n                \"headline\": \"Gale Warning issued December 3 at 4:00AM AKST until December 3 at 5:00PM AKST by NWS Anchorage AK\",\n                \"description\": \"Coastal Waters Forecast for Southwest Alaska+Bristol Bay+The\\nAlaska Peninsula Waters and the Aleutian Islands up to 100 nm out.\\n\\nWind forecasts reflect the predominant speed and direction\\nexpected. Sea forecasts represent an average of the highest\\none-third of the combined wind wave and swell height.\\n\\n.TODAY...N wind 40 kt. Seas 26 ft.\\n.TONIGHT...NE wind 30 kt. Seas 20 ft.\\n.THU...E wind 20 kt increasing to 30 kt in the afternoon. Seas\\n14 ft.\\n.THU NIGHT...SE wind 30 kt. Seas 10 ft.\\n.FRI...NE wind 20 kt. Seas 10 ft.\\n.SAT...NE wind 25 kt. Seas 9 ft.\\n.SUN...NE wind 25 kt. Seas 17 ft.\",\n                \"instruction\": null,\n                \"response\": \"Avoid\",\n                \"parameters\": {\n                    \"AWIPSidentifier\": [\n                        \"CWFALU\"\n                    ],\n                    \"WMOidentifier\": [\n                        \"FZAK52 PAFC 031300\"\n                    ],\n                    \"NWSheadline\": [\n                        \"GALE WARNING TODAY\"\n                    ],\n                    \"BLOCKCHANNEL\": [\n                        \"EAS\",\n                        \"NWEM\",\n                        \"CMAS\"\n                    ],\n                    \"VTEC\": [\n                        \"/O.NEW.PAFC.GL.W.5660.251203T1400Z-251204T0200Z/\"\n                    ],\n                    \"eventEndingTime\": [\n                        \"2025-12-03T17:00:00-09:00\"\n                    ]\n                },\n                \"scope\": \"Public\",\n                \"code\": \"IPAWSv1.0\",\n                \"language\": \"en-US\",\n                \"web\": \"http://www.weather.gov\",\n                \"eventCode\": {\n                    \"SAME\": [\n                        \"NWS\"\n                    ],\n                    \"NationalWeatherService\": [\n                        \"GLW\"\n                    ]\n                }\n            }\n        },\n        {\n            \"id\": \"https://api.weather.gov/alerts/urn:oid:2.49.0.1.840.0.16ee1729296b80b5948b72c512c8722f6075ae6c.036.1\",\n            \"type\": \"Feature\",\n            \"geometry\": null,\n            \"properties\": {\n                \"@id\": \"https://api.weather.gov/alerts/urn:oid:2.49.0.1.840.0.16ee1729296b80b5948b72c512c8722f6075ae6c.036.1\",\n                \"@type\": \"wx:Alert\",\n                \"id\": \"urn:oid:2.49.0.1.840.0.16ee1729296b80b5948b72c512c8722f6075ae6c.036.1\",\n                \"areaDesc\": \"Saint Matthew Island Waters\",\n                \"geocode\": {\n                    \"SAME\": [\n                        \"058767\"\n                    ],\n                    \"UGC\": [\n                        \"PKZ767\"\n                    ]\n                },\n                \"affectedZones\": [\n                    \"https://api.weather.gov/zones/forecast/PKZ767\"\n                ],\n                \"references\": [],\n                \"sent\": \"2025-12-03T04:00:00-09:00\",\n                \"effective\": \"2025-12-03T04:00:00-09:00\",\n                \"onset\": \"2025-12-03T04:00:00-09:00\",\n                \"expires\": \"2025-12-03T17:00:00-09:00\",\n                \"ends\": \"2025-12-04T05:00:00-09:00\",\n                \"status\": \"Actual\",\n                \"messageType\": \"Alert\",\n                \"category\": \"Met\",\n                \"severity\": \"Moderate\",\n                \"certainty\": \"Likely\",\n                \"urgency\": \"Expected\",\n                \"event\": \"Gale Warning\",\n                \"sender\": \"w-nws.webmaster@noaa.gov\",\n                \"senderName\": \"NWS Anchorage AK\",\n                \"headline\": \"Gale Warning issued December 3 at 4:00AM AKST until December 4 at 5:00AM AKST by NWS Anchorage AK\",\n                \"description\": \"Coastal Waters Forecast for Southwest Alaska+Bristol Bay+The\\nAlaska Peninsula Waters and the Aleutian Islands up to 100 nm out.\\n\\nWind forecasts reflect the predominant speed and direction\\nexpected. Sea forecasts represent an average of the highest\\none-third of the combined wind wave and swell height.\\n\\n.TODAY...N wind 40 kt E of Saint Matthew Island...N 35 kt W of\\nSaint Matthew Island. Seas 16 ft. Freezing spray.\\n.TONIGHT...NE wind 35 kt. Seas 12 ft. Freezing spray.\\n.THU...NE wind 30 kt E of Saint Matthew Island...E 25 kt W of\\nSaint Matthew Island. Seas 7 ft.\\n.THU NIGHT...E wind 25 kt. Seas 7 ft.\\n.FRI...E wind 25 kt. Seas 9 ft.\\n.SAT...NE wind 30 kt. Seas 13 ft.\\n.SUN...NE wind 35 kt. Seas 15 ft.\",\n                \"instruction\": null,\n                \"response\": \"Avoid\",\n                \"parameters\": {\n                    \"AWIPSidentifier\": [\n                        \"CWFALU\"\n                    ],\n                    \"WMOidentifier\": [\n                        \"FZAK52 PAFC 031300\"\n                    ],\n                    \"NWSheadline\": [\n                        \"GALE WARNING THROUGH TONIGHT\"\n                    ],\n                    \"BLOCKCHANNEL\": [\n                        \"EAS\",\n                        \"NWEM\",\n                        \"CMAS\"\n                    ],\n                    \"VTEC\": [\n                        \"/O.NEW.PAFC.GL.W.5671.251203T1300Z-251204T1400Z/\"\n                    ],\n                    \"eventEndingTime\": [\n                        \"2025-12-04T05:00:00-09:00\"\n                    ]\n                },\n                \"scope\": \"Public\",\n                \"code\": \"IPAWSv1.0\",\n                \"language\": \"en-US\",\n                \"web\": \"http://www.weather.gov\",\n                \"eventCode\": {\n                    \"SAME\": [\n                        \"NWS\"\n                    ],\n                    \"NationalWeatherService\": [\n                        \"GLW\"\n                    ]\n                }\n            }\n        },\n        {\n            \"id\": \"https://api.weather.gov/alerts/urn:oid:2.49.0.1.840.0.16ee1729296b80b5948b72c512c8722f6075ae6c.010.1\",\n            \"type\": \"Feature\",\n            \"geometry\": null,\n            \"properties\": {\n                \"@id\": \"https://api.weather.gov/alerts/urn:oid:2.49.0.1.840.0.16ee1729296b80b5948b72c512c8722f6075ae6c.010.1\",\n                \"@type\": \"wx:Alert\",\n                \"id\": \"urn:oid:2.49.0.1.840.0.16ee1729296b80b5948b72c512c8722f6075ae6c.010.1\",\n                \"areaDesc\": \"Nelson Lagoon to Cape Sarichef out to 15 NM\",\n                \"geocode\": {\n                    \"SAME\": [\n                        \"058758\"\n                    ],\n                    \"UGC\": [\n                        \"PKZ758\"\n                    ]\n                },\n                \"affectedZones\": [\n                    \"https://api.weather.gov/zones/forecast/PKZ758\"\n                ],\n                \"references\": [],\n                \"sent\": \"2025-12-03T04:00:00-09:00\",\n                \"effective\": \"2025-12-03T04:00:00-09:00\",\n                \"onset\": \"2025-12-03T04:00:00-09:00\",\n                \"expires\": \"2025-12-03T17:00:00-09:00\",\n                \"ends\": \"2025-12-04T17:00:00-09:00\",\n                \"status\": \"Actual\",\n                \"messageType\": \"Alert\",\n                \"category\": \"Met\",\n                \"severity\": \"Minor\",\n                \"certainty\": \"Likely\",\n                \"urgency\": \"Expected\",\n                \"event\": \"Small Craft Advisory\",\n                \"sender\": \"w-nws.webmaster@noaa.gov\",\n                \"senderName\": \"NWS Anchorage AK\",\n                \"headline\": \"Small Craft Advisory issued December 3 at 4:00AM AKST until December 4 at 5:00PM AKST by NWS Anchorage AK\",\n                \"description\": \"Coastal Waters Forecast for Southwest Alaska+Bristol Bay+The\\nAlaska Peninsula Waters and the Aleutian Islands up to 100 nm out.\\n\\nWind forecasts reflect the predominant speed and direction\\nexpected. Sea forecasts represent an average of the highest\\none-third of the combined wind wave and swell height.\\n\\n.TODAY...E wind 25 kt. Seas 7 ft. Rain showers.\\n.TONIGHT...NE wind 20 kt. Seas 10 ft. Rain showers.\\n.THU...NE wind 20 kt. Seas 9 ft.\\n.THU NIGHT...NE wind 20 kt. Seas 7 ft.\\n.FRI...NE wind 25 kt. Seas 9 ft.\\n.SAT...N wind 40 kt. Seas 15 ft.\\n.SUN...N wind 30 kt. Seas 13 ft.\",\n                \"instruction\": null,\n                \"response\": \"Avoid\",\n                \"parameters\": {\n                    \"AWIPSidentifier\": [\n                        \"CWFALU\"\n                    ],\n                    \"WMOidentifier\": [\n                        \"FZAK52 PAFC 031300\"\n                    ],\n                    \"NWSheadline\": [\n                        \"SMALL CRAFT ADVISORY THROUGH THURSDAY\"\n                    ],\n                    \"BLOCKCHANNEL\": [\n                        \"EAS\",\n                        \"NWEM\",\n                        \"CMAS\"\n                    ],\n                    \"VTEC\": [\n                        \"/O.NEW.PAFC.SC.Y.5645.251203T1300Z-251205T0200Z/\"\n                    ],\n                    \"eventEndingTime\": [\n                        \"2025-12-04T17:00:00-09:00\"\n                    ]\n                },\n                \"scope\": \"Public\",\n                \"code\": \"IPAWSv1.0\",\n                \"language\": \"en-US\",\n                \"web\": \"http://www.weather.gov\",\n                \"eventCode\": {\n                    \"SAME\": [\n                        \"NWS\"\n                    ],\n                    \"NationalWeatherService\": [\n                        \"SCY\"\n                    ]\n                }\n            }\n        },\n        {\n            \"id\": \"https://api.weather.gov/alerts/urn:oid:2.49.0.1.840.0.16ee1729296b80b5948b72c512c8722f6075ae6c.019.1\",\n            \"type\": \"Feature\",\n            \"geometry\": null,\n            \"properties\": {\n                \"@id\": \"https://api.weather.gov/alerts/urn:oid:2.49.0.1.840.0.16ee1729296b80b5948b72c512c8722f6075ae6c.019.1\",\n                \"@type\": \"wx:Alert\",\n                \"id\": \"urn:oid:2.49.0.1.840.0.16ee1729296b80b5948b72c512c8722f6075ae6c.019.1\",\n                \"areaDesc\": \"Nikolski to Seguam Pacfic Side out to 15 NM\",\n                \"geocode\": {\n                    \"SAME\": [\n                        \"058777\"\n                    ],\n                    \"UGC\": [\n                        \"PKZ777\"\n                    ]\n                },\n                \"affectedZones\": [\n                    \"https://api.weather.gov/zones/forecast/PKZ777\"\n                ],\n                \"references\": [],\n                \"sent\": \"2025-12-03T04:00:00-09:00\",\n                \"effective\": \"2025-12-03T04:00:00-09:00\",\n                \"onset\": \"2025-12-03T05:00:00-09:00\",\n                \"expires\": \"2025-12-03T17:00:00-09:00\",\n                \"ends\": \"2025-12-03T17:00:00-09:00\",\n                \"status\": \"Actual\",\n                \"messageType\": \"Alert\",\n                \"category\": \"Met\",\n                \"severity\": \"Moderate\",\n                \"certainty\": \"Likely\",\n                \"urgency\": \"Expected\",\n                \"event\": \"Gale Warning\",\n                \"sender\": \"w-nws.webmaster@noaa.gov\",\n                \"senderName\": \"NWS Anchorage AK\",\n                \"headline\": \"Gale Warning issued December 3 at 4:00AM AKST until December 3 at 5:00PM AKST by NWS Anchorage AK\",\n                \"description\": \"Coastal Waters Forecast for Southwest Alaska+Bristol Bay+The\\nAlaska Peninsula Waters and the Aleutian Islands up to 100 nm out.\\n\\nWind forecasts reflect the predominant speed and direction\\nexpected. Sea forecasts represent an average of the highest\\none-third of the combined wind wave and swell height.\\n\\n.TODAY...N wind 35 kt. Seas 20 ft.\\n.TONIGHT...N wind 30 kt. Seas 19 ft.\\n.THU...N wind 30 kt. Seas 14 ft.\\n.THU NIGHT...N wind 20 kt. Seas 9 ft.\\n.FRI...E wind 20 kt. Seas 6 ft.\\n.SAT...N wind 25 kt. Seas 9 ft.\\n.SUN...N wind 30 kt. Seas 18 ft.\"
